vi "onHttpGet.vi"(8 "error in":errorcluster, 10 "httpRequest":refnum<class "httpRequest.lvclass">, 11 "advanced-http-client in":refnum<class "advanced-http-client.lvclass">) -> (0 "error out":errorcluster, 2 "httpResponse":refnum<class "httpResponse.lvclass">, 3 "advanced-http-client out":refnum<class "advanced-http-client.lvclass">)   [LabVIEW 2020, in "HttpClient.NiAdvanced.lvlib" / "advanced-http-client.lvclass"]
uses:
  advanced-http-client.lvclass
  advanced-http-client.lvclass/advanced-http-client.ctl
  <vilib>/NI/Advanced HTTP Client/Session.lvclass
  http-client-pkg/httpRequest/httpRequest.lvclass
  http-client-pkg/httpResponse/httpResponse.lvclass
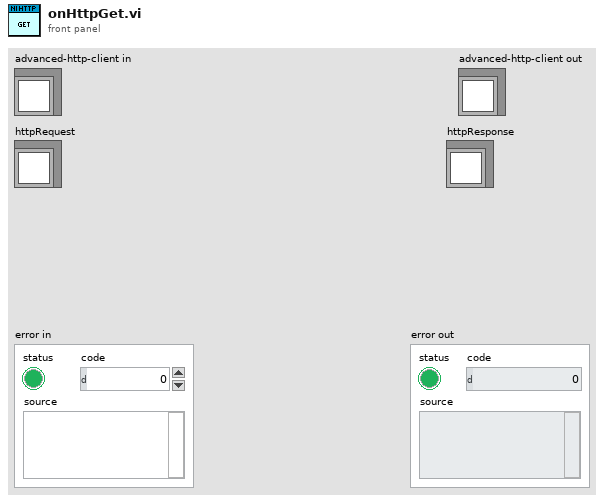
[diagram p1: front panel]
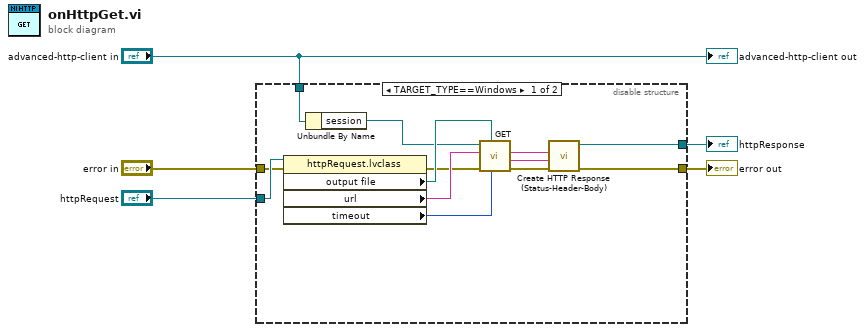
[diagram p0: block diagram]
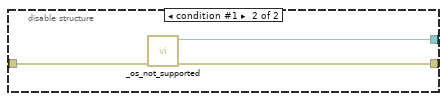
[diagram p2: hidden frame]
diagram:
  n1 = disable-structure shown="TARGET_TYPE==Windows" {
    disable-tunnel: "error in" -> [w13 w21]
    disable-tunnel: [w7 w20] -> w4
    disable-tunnel: [w6 w19] -> w3
    disable-tunnel: "httpRequest" -> [w18 _]
    disable-tunnel: "advanced-http-client in" -> [w12 _]
    frame condition #0 (active) {
      n2 = property class="httpRequest.lvclass"(reference=w18, error in=w13) -> (error out=w14:errorcluster, "output file"=w17:path, "url"=w16:string, "timeout"=w15:i32)  [unwired: 1 out]
      n3 = Unbundle By Name(w12) -> ("session"=w11:refnum<class "Session.lvclass">)
      n4 = call <vilib>:"GET.vi"("timeout"=w15, "output file"=w17, "error in"=w14, "url"=w16, "session in"=w11) -> ("error out"=w8:errorcluster, "body"=w10:string, "headers"=w9:string)  [unwired: 2 in, 2 out]
      n5 = call "Create HTTP Response (Status-Header-Body).vi"("error in"=w8, "body"=w10, "Headers w/ status line(s)"=w9) -> ("error out"=w7:errorcluster, "httpResponse out"=w6:refnum<class "httpResponse.lvclass">)  [unwired: 7 in]
    }
    frame condition #1 {
      n6 = call "_os_not_supported.vi"("error in (no error)"=w21) -> ("error out"=w20:errorcluster, "httpResponse"=w19:refnum<class "httpResponse.lvclass">)  [unwired: 9 in]
    }
  }
  "error out" <- w4
  "httpResponse" <- w3
  "advanced-http-client out" <- "advanced-http-client in"
